vi "Wait on Running.vi"(7 "Timeout (2000ms)":i32=2000, 8 "error in (no error)":errorcluster, 10 "Value":bool, 11 "2DArrayManager in":refnum<class "2DArrayManager.lvclass">) -> (0 "error out":errorcluster, 3 "2DArrayManager out":refnum<class "2DArrayManager.lvclass">)   [LabVIEW 2020, in "OOPanel.lvlib" / "2DArrayManager.lvclass"]
uses:
  2DArrayManager.lvclass
  2DArrayManager.lvclass/2DArrayManager.ctl
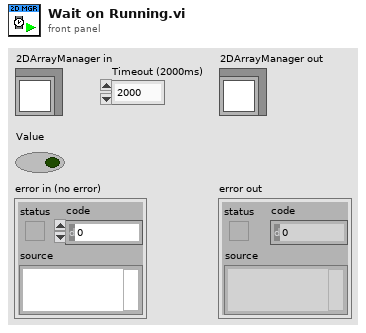
[diagram p1: front panel]
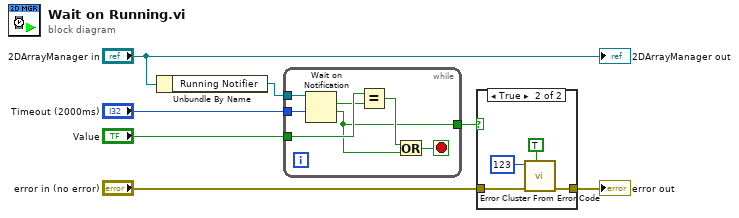
[diagram p0: block diagram]
diagram:
  n1 = Unbundle By Name("2DArrayManager in") -> ("Running Notifier"=w7:refnum<notifier>)
  n2 = while {
    tunnel: w7 -> [w14]
    tunnel: "Timeout (2000ms)" -> [w13]
    tunnel: "Value" -> [w12]
    tunnel: [w8] -> w3
    stop <- w10 stop-if-true
    n3 = Wait on Notification(notifier=w14, timeout in ms (-1)=w13) -> (notification=w9:bool, timed out?=w8:bool)  [unwired: 2 in, 2 out]
    n4 = Equal?(x=w12, y=w9) -> (x = y?=w11:bool)
    n5 = Or(x=w11, y=w8) -> (x .or. y?=w10:bool)
  }
  n6 = case shown="True" w3 {
    tunnel: "error in (no error)" -> [w15 w19]
    tunnel: [w15 w16] -> w1
    frame False {
    }
    frame True {
      n7 = call <vilib>:"Error Cluster From Error Code.vi"("show call chain? (False)"=TRUE, "error in (no error)"=w19, "error code (0)"=123) -> ("error out"=w16:errorcluster)  [unwired: 6 in]
    }
  }
  "error out" <- w1
  "2DArrayManager out" <- "2DArrayManager in"
